vi "to string.vi"(8 "error in":errorcluster, 11 "io configuration in":refnum<class "io configuration.lvclass">) -> (0 "error out":errorcluster, 1 "data":string, 2 "version":string, 3 "io configuration out":refnum<class "io configuration.lvclass">)   [LabVIEW 2015, in "io configuration.lvclass"]
doc: "Provides an interface for saving a module configuration to a file or other serialized data source. It is recommended that all children of this class store data in two sets--data required for its own initialization, and any data required for parent initialization--and that each implementation uses the <b>Call Parent Method</b> primitive to serialize parent information."
uses:
  io configuration.lvclass
  <vilib>/NI/Tag Bus/tag/Data Type.ctl
  fpga resource supported data types.ctl
  io configuration.lvclass/io configuration.ctl
  fifo channel/fifo channel.lvclass
  <vilib>/NI/Tag Bus/tag/tag descriptor.lvclass/tag descriptor.ctl
  fpga channel/fpga channel.lvclass/fpga channel.ctl
  <vilib>/NI/Tag Bus/tag/read tag name.vi
  <vilib>/NI/Tag Bus/tag/read data type.vi
  fpga channel/Read fpga res type.vi
  <vilib>/NI/Tag Bus Module Framework/module configuration/TBM module configuration.lvclass
  <vilib>/NI/Tag Bus Module Framework/channel/TBM channel.lvclass
  <vilib>/NI/Configuration Framework/serializable configuration/NISE_CEF_serializable configuration.lvclass
  <vilib>/NI/Tag Bus/tag/tag descriptor.lvclass
panel:
  out "fpga type":T1[](array[typedef])
  out "fifo?":bool[](array[boolean])
  out "Data Type":T2[](array[typedef])
  out "Name":string[](array[string])
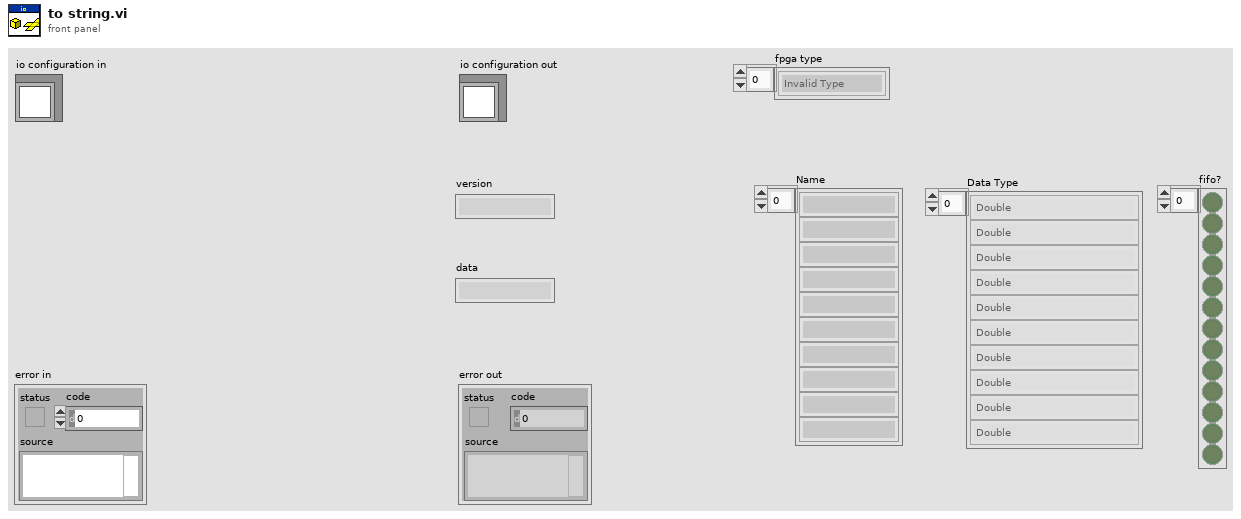
[diagram p1: front panel]
types:
  T1 = typedef "io configuration.lvclass/fpga resource supported data types.ctl" = enum16{"Invalid Type", "Single", "I64", "I32", "I16", "I8", "U64", "U32", "U16", "U8", "Boolean", "FXP I,20,5", "FXP I,24,5", "FXP I,24,10", "Fifo 1023,I16"}
  T2 = typedef "tag bus.lvlib/tag descriptor.lvclass/Data Type.ctl" = enum16{"Double", "Single", "I64", "I32", "I16", "I8", "U64", "U32", "U16", "U8", "Boolean", "String", "Array of Double", "Array of Single", "Array of I64", "Array of I32", "Array of I16", "Array of I8", "Array of U64", "Array of U32", "Array of U16", "Array of U8", "Array of Boolean", "Array of String"}
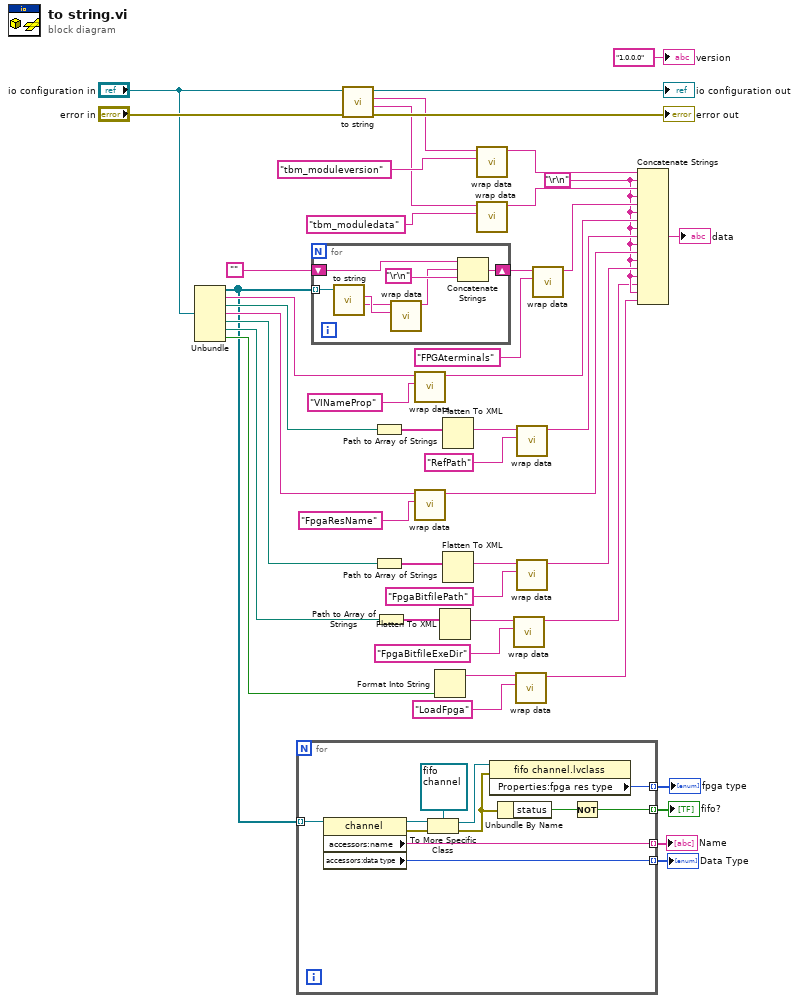
[diagram p0: block diagram]
diagram:
  w11 = "\r\n"
  n1 = Unbundle("io configuration in") -> (w5:refnum<class "TBM channel.lvclass">[], w25:string, w24:path, w22:string, w16:path, w7:path, w9:bool)
  n2 = for {
    tunnel: w5 -> [w58] mode=indexing
    tunnel: [w56] -> w4 mode=indexing
    tunnel: [w55] -> w3 mode=indexing
    tunnel: [w50] -> w2 mode=indexing
    tunnel: [w48] -> w1 mode=indexing
    n3 = property class="channel"(reference=w58) -> (reference out=w54:refnum<class "TBM channel.lvclass">, error out=w57:errorcluster, "accessors:name"=w56:string, "accessors:data type"=w55:T2)  [unwired: 1 in]
    n4 = To More Specific Class(target class=refnum<class "fifo channel.lvclass"> refnum ("fifo channel.lvclass"), reference=w54, error in=w57) -> (specific class reference=w53:refnum<class "fifo channel.lvclass">, error out=w52:errorcluster)
    n5 = property class="fifo channel.lvclass"(reference=w53, error in=w52) -> ("Properties:fpga res type"=w48:T1)  [unwired: 2 out]
    n6 = Unbundle By Name(w52) -> ("status"=w51:bool)
    n7 = Not(x=w51) -> (.not. x?=w50:bool)
  }
  "Name" <- w4
  "Data Type" <- w3
  "fifo?" <- w2
  "fpga type" <- w1
  n8 = for {
    tunnel: w5 -> [w61] mode=indexing
    shift-right: [w64] -> w33
    shift-left: "" -> [w63]
    n9 = call-dynamic "to string.vi"("channel in"=w61) -> ("channel data"=w59:string, "identifier"=w60:string)  [unwired: 7 in, 2 out]
    n10 = call <vilib>:"wrap data.vi"("identifier"=w60, "data to wrap"=w59) -> ("wrapped data"=w62:string)  [unwired: 9 in]
    n11 = Concatenate Strings(w63, w62, "\r\n") -> (w64:string)
  }
  n12 = call-parent "to string.vi"("error in"="error in", "module configuration in"="io configuration in") -> ("error out"=→"error out":errorcluster, "data"=w39:string, "version"=w40:string, "module configuration out"=→"io configuration out":refnum<class "io configuration.lvclass">)  [unwired: 6 in]
  n13 = Path to Array of Strings(0:w24) -> (2:w28:string[])  [unwired: 1 out]
  n14 = Path to Array of Strings(0:w16) -> (2:w19:string[])  [unwired: 1 out]
  n15 = Path to Array of Strings(0:w7) -> (2:w6:string[])  [unwired: 1 out]
  n16 = call <vilib>:"wrap data.vi"("identifier"="VINameProp" ("additional identifier"), "data to wrap"=w25) -> ("wrapped data"=w26:string)  [unwired: 9 in]
  n17 = call <vilib>:"wrap data.vi"("identifier"="FpgaResName" ("additional identifier"), "data to wrap"=w22) -> ("wrapped data"=w21:string)  [unwired: 9 in]
  n18 = Format Into String(w9) -> (resulting string=w12:string)  [unwired: 3 in, 1 out]
  n19 = Flatten To XML(anything=w6) -> (xml string=w14:string)
  n20 = Flatten To XML(anything=w28) -> (xml string=w27:string)
  n21 = Flatten To XML(anything=w19) -> (xml string=w20:string)
  n22 = call <vilib>:"wrap data.vi"("identifier"="tbm_moduleversion" ("additional identifier"), "data to wrap"=w40) -> ("wrapped data"=w42:string)  [unwired: 9 in]
  n23 = call <vilib>:"wrap data.vi"("identifier"="tbm_moduledata" ("additional identifier"), "data to wrap"=w39) -> ("wrapped data"=w41:string)  [unwired: 9 in]
  n24 = call <vilib>:"wrap data.vi"("identifier"="FpgaBitfileExeDir" ("additional identifier"), "data to wrap"=w14) -> ("wrapped data"=w10:string)  [unwired: 9 in]
  n25 = call <vilib>:"wrap data.vi"("identifier"="LoadFpga" ("additional identifier"), "data to wrap"=w12) -> ("wrapped data"=w8:string)  [unwired: 9 in]
  n26 = call <vilib>:"wrap data.vi"("identifier"="RefPath" ("additional identifier"), "data to wrap"=w27) -> ("wrapped data"=w30:string)  [unwired: 9 in]
  n27 = call <vilib>:"wrap data.vi"("identifier"="FpgaBitfilePath" ("additional identifier"), "data to wrap"=w20) -> ("wrapped data"=w17:string)  [unwired: 9 in]
  n28 = call <vilib>:"wrap data.vi"("identifier"="FPGAterminals" ("additional identifier"), "data to wrap"=w33) -> ("wrapped data"=w36:string)  [unwired: 9 in]
  n29 = Concatenate Strings(w42, w11, w41, w11, w36, w11, w26, w11, w30, w11, w21, w11, w17, w11, w10, w11, w8) -> (→"data":string)
  "version" <- "1.0.0.0" ("version")
